vi "SetProcessGraphs(SubVI).vi"(1 "Blue":refnum<vi>, 2 "Red":refnum<vi>) -> ()   [LabVIEW 2013, in "main.lvlib"]
uses:
  main.lvlib
  <vilib>/Utility/miscctls.llb/LVPositionTypeDef.ctl
  <vilib>/Utility/miscctls.llb/LVRectTypeDef.ctl
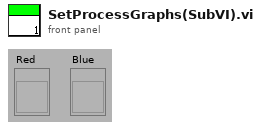
[diagram p1: front panel]
types:
  T1 = typedef "LVPositionTypeDef.ctl" = cluster{"Left":i32, "Top":i32}
  T2 = typedef "LVRectTypeDef.ctl" = cluster{"Left":i16, "Top":i16, "Right":i16, "Bottom":i16}
  T3 = typedef "LVBoundsTypeDef.ctl" = cluster{"Width":u32, "Height":u32}
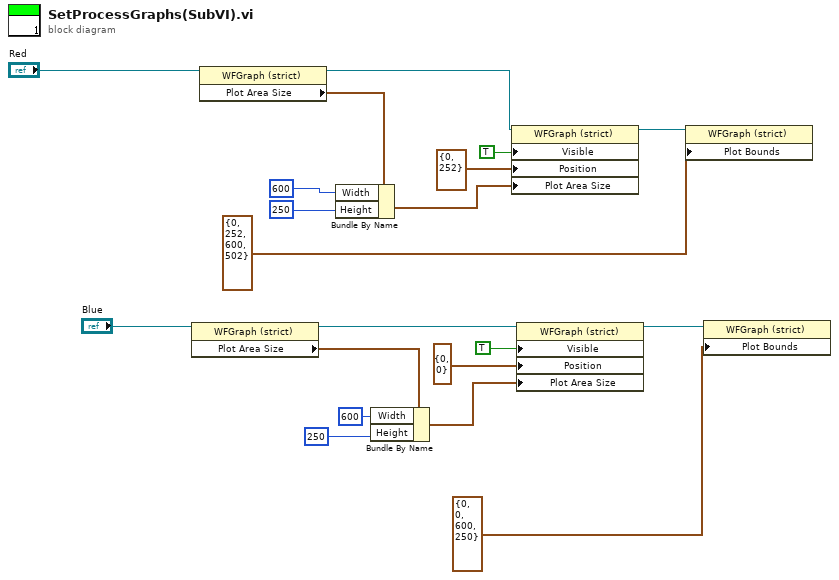
[diagram p0: block diagram]
diagram:
  n1 = property class="WFGraph (strict)"(reference="Blue") -> (reference out=w10:refnum<vi>, "Plot Area Size"=w9:T3)  [unwired: 1 in, 1 out]
  n2 = property class="WFGraph (strict)"(reference="Red") -> (reference out=w4:refnum<vi>, "Plot Area Size"=w5:T3)  [unwired: 1 in, 1 out]
  n3 = Bundle By Name(cluster=w5, "Width"=u32 600, "Height"=u32 250) -> (w12:T3)
  n4 = Bundle By Name(cluster=w9, "Width"=u32 600, "Height"=u32 250) -> (w11:T3)
  n5 = property class="WFGraph (strict)"(reference=w4, "Visible"=TRUE, "Position"=T1 {"Left"=0, "Top"=252}, "Plot Area Size"=w12) -> (reference out=w17:refnum<vi>)  [unwired: 1 in, 1 out]
  n6 = property class="WFGraph (strict)"(reference=w10, "Visible"=TRUE ("x"), "Position"=T1 {"Left"=0, "Top"=0}, "Plot Area Size"=w11) -> (reference out=w19:refnum<vi>)  [unwired: 1 in, 1 out]
  n7 = property class="WFGraph (strict)"(reference=w17, "Plot Bounds"=T2 {"Left"=0, "Top"=252, "Right"=600, "Bottom"=502} ("Plot Area Bounds")) -> ()  [unwired: 1 in, 2 out]
  n8 = property class="WFGraph (strict)"(reference=w19, "Plot Bounds"=T2 {"Left"=0, "Top"=0, "Right"=600, "Bottom"=250} ("Plot Area Bounds")) -> ()  [unwired: 1 in, 2 out]
